vi "Write destiny.vi"(8 "error in (no error)":errorcluster, 10 "destiny":dbl[](array[numeric]), 11 "GoToSkill_v2 in":refnum<class "GoToSkill_v2.lvclass">) -> (0 "error out":errorcluster, 3 "GoToSkill_v2 out":refnum<class "GoToSkill_v2.lvclass">)   [LabVIEW 2023, in "GoToSkill_v2.lvclass"]
uses:
  GoToSkill_v2.lvclass
  GoToSkill_v2.lvclass/GoToSkill_v2.ctl
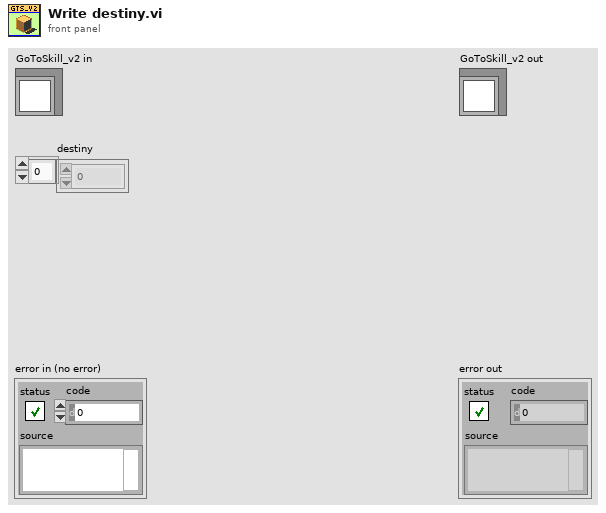
[diagram p1: front panel]
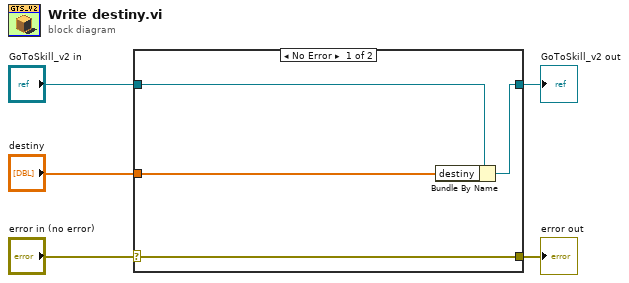
[diagram p0: block diagram]
diagram:
  n1 = case shown="No Error" "error in (no error)" {
    selector: "error in (no error)" -> [w9 w10]
    tunnel: [w9 w10] -> w4
    tunnel: [w7 w11] -> w2
    tunnel: "GoToSkill_v2 in" -> [w8 w11]
    tunnel: "destiny" -> [w6 _]
    frame No Error {
      n2 = Bundle By Name(cluster=w8, "destiny"=w6) -> (w7:refnum<class "GoToSkill_v2.lvclass">)
    }
    frame Error {
    }
  }
  "error out" <- w4
  "GoToSkill_v2 out" <- w2
